vi "PutToList.vi"(4 "Wyjœcie_Exceed":string[][](array[string]), 6 "Wejscie_Exceed":string[][](array[string]), 11 "Previous":string[][](array[string])) -> (3 "Next":string[][](array[string]))   [LabVIEW 2021]
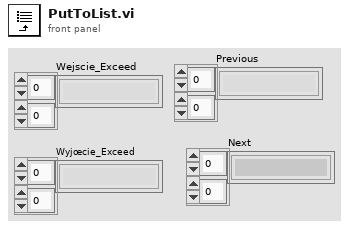
[diagram p1: front panel]
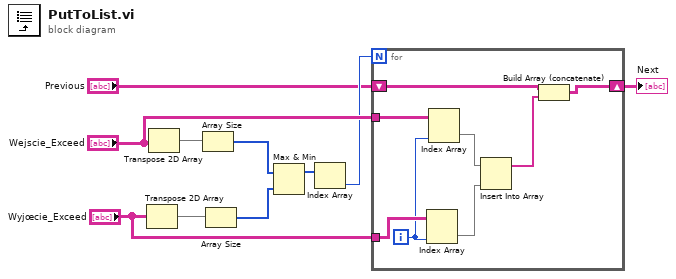
[diagram p0: block diagram]
diagram:
  n1 = Transpose 2D Array(2D array="Wyjœcie_Exceed") -> (transposed array=w9:string[][])
  n2 = Transpose 2D Array(2D array="Wejscie_Exceed") -> (transposed array=w10:string[][])
  n3 = Array Size(array=w10) -> (size(s)=w8:i32[])
  n4 = Array Size(array=w9) -> (size(s)=w7:i32[])
  n5 = Max & Min(x=w8, y=w7) -> (max(x,y)=w6:i32[])  [unwired: 1 out]
  n6 = Index Array(array=w6) -> (element=w4:i32)  [unwired: 1 in]
  n7 = for {
    N: w4 -> [_]
    tunnel: "Wejscie_Exceed" -> [w18]
    tunnel: "Wyjœcie_Exceed" -> [w17]
    shift-right: [w13] -> w1
    shift-left: "Previous" -> [w12]
    i -> [w11]
    n8 = Index Array(array=w17, index (col)=w11) -> (element=w15:string[])  [unwired: 1 in]
    n9 = Index Array(array=w18, index (col)=w11) -> (element=w16:string[])  [unwired: 1 in]
    n10 = Insert Into Array(array=w16, new element=w15) -> (w14:string[])  [unwired: 1 in]
    n11 = Build Array (concatenate)(w12, w14) -> (w13:string[][])
  }
  "Next" <- w1
